vi "Get RT INI location.vi"(8 "error in (no error)":errorcluster, 11 "RT Management in":refnum<class "RT Management.lvclass">) -> (0 "error out":errorcluster, 2 "RT INI Location":string, 3 "RT Management out":refnum<class "RT Management.lvclass">)   [LabVIEW 2015, in "RT Management.lvlib" / "RT Management.lvclass"]
doc: "Gets the RT INI (ni-rt.ini) path based upon the target's OS."
uses:
  RT Management.lvclass
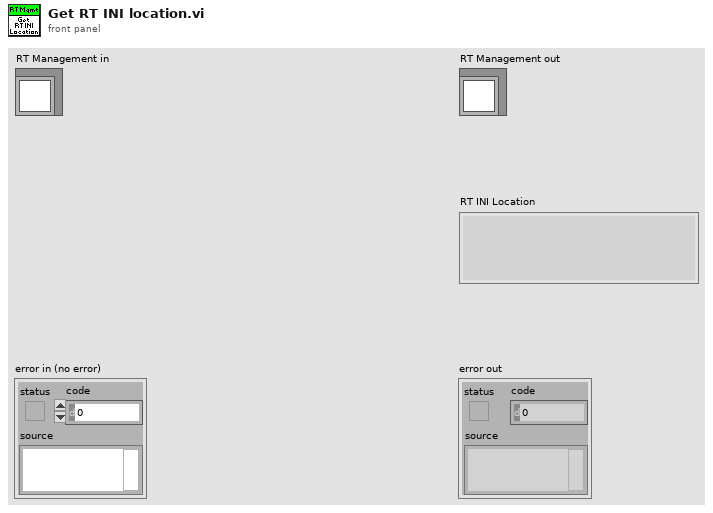
[diagram p1: front panel]
types:
  T1 = typedef "RT Management.lvlib/RT Management.lvclass/Operating system.ctl" = enum16{"Unknown", "VxWorks", "PharLap", "Linux-ARM", "Linux-x64"}
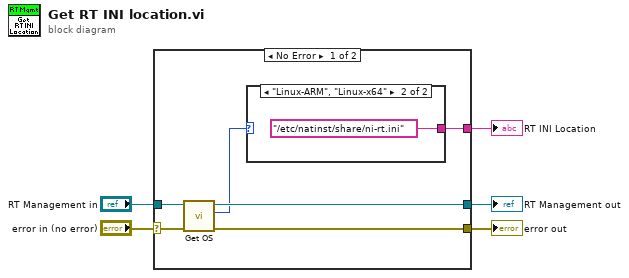
[diagram p0: block diagram]
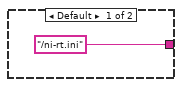
[diagram p2: hidden frame]
diagram:
  n1 = case shown="No Error" "error in (no error)" {
    selector: "error in (no error)" -> [w10 w15]
    tunnel: [w9 w15] -> w4
    tunnel: [w7 w14] -> w2
    tunnel: "RT Management in" -> [w8 w14]
    tunnel: [w11 _] -> w1
    frame No Error {
      n2 = call "Get OS.vi"("error in (no error)"=w10, "RT Management in"=w8) -> ("error out"=w9:errorcluster, "Operating System"=w6:T1, "RT Management out"=w7:refnum<class "RT Management.lvclass">)  [unwired: 6 in, 1 out]
      n3 = case shown="\"Linux-ARM\", \"Linux-x64\"" w6 {
        tunnel: ["/ni-rt.ini" ("Remote path") "/etc/natinst/share/ni-rt.ini" ("Remote path")] -> w11
        frame Default {
        }
        frame "Linux-ARM", "Linux-x64" {
        }
      }
    }
    frame Error {
    }
  }
  "error out" <- w4
  "RT Management out" <- w2
  "RT INI Location" <- w1
